vi "HandleAbort.vi"(8 "error in (no error)":errorcluster, 11 "Acquisition in":refnum<class "Acquisition.lvclass">) -> (0 "error out":errorcluster, 2 "abort?":bool, 3 "Acquisition out":refnum<class "Acquisition.lvclass">)   [LabVIEW 2018, in "Acquisition.lvclass"]
uses:
  Acquisition.lvclass
  C:/Users/devstaff/sparc4/s4gui/Versao ZeroMQ REQ-REP/SPARC4_GUI -v1.0.0/Server/Server.lvclass
  Server/Server.lvclass/Server.ctl
  Acquisition.lvclass/Acquisition.ctl
  Channel/Channel.lvclass
  StateMachine/State Machine.lvclass
  Server/Server.lvclass
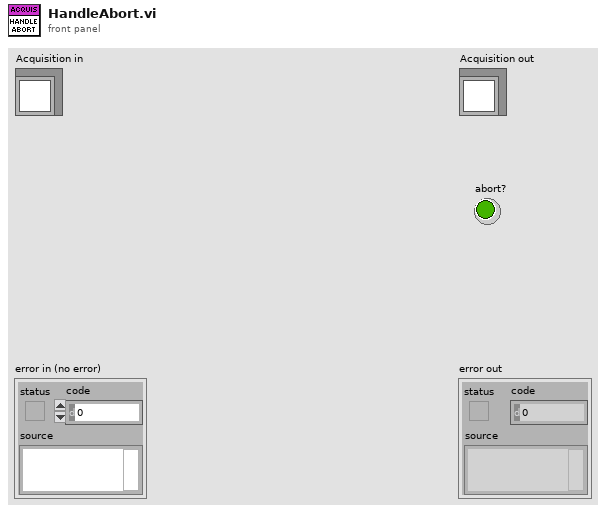
[diagram p1: front panel]
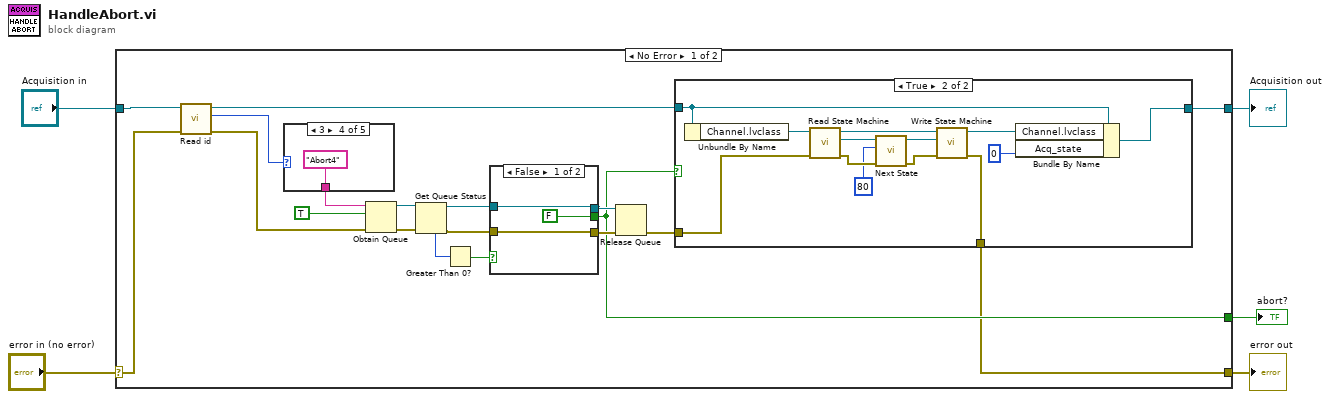
[diagram p0: block diagram]
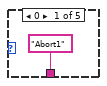
[diagram p2: hidden frame]
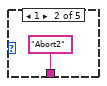
[diagram p3: hidden frame]
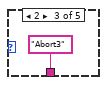
[diagram p4: hidden frame]
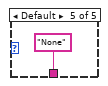
[diagram p5: hidden frame]
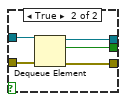
[diagram p7: hidden frame]
diagram:
  n1 = case shown="No Error" "error in (no error)" {
    selector: "error in (no error)" -> [w7 w54]
    tunnel: [w8 w54] -> w4
    tunnel: [w24 w53] -> w2
    tunnel: "Acquisition in" -> [w23 w53]
    tunnel: [w11 _] -> w1
    frame No Error {
      n2 = call "Read id.vi"("error in (no error)"=w7, "Server in"=w23) -> ("error out"=w6:errorcluster, "id"=w10:u32, "Server out"=w22:refnum<class "Acquisition.lvclass">)  [unwired: 7 in]
      n3 = case shown="3" w10 {
        tunnel: ["Abort1" ("name (unnamed)") "Abort2" ("name (unnamed)") "Abort3" ("name (unnamed)") "Abort4" ("name (unnamed)") "None" ("name (unnamed)")] -> w21
        frame 0 {
        }
        frame 1 {
        }
        frame 2 {
        }
        frame 3 {
        }
        frame Default {
        }
      }
      n4 = Obtain Queue(name (unnamed)=w21, element data type=TRUE, error in (no error)=w6) -> (queue out=w18:refnum<queue>, error out=w19:errorcluster)  [unwired: 2 in, 1 out]
      n5 = Get Queue Status(queue=w18, error in (no error)=w19) -> (queue out=w15:refnum<queue>, error out=w14:errorcluster, # elements in queue=w17:i32)  [unwired: 1 in, 5 out]
      n6 = Greater Than 0?(x=w17) -> (x > 0?=w16:bool)
      n7 = case shown="False" w16 {
        tunnel: w15 -> [w46 w51]
        tunnel: w14 -> [w45 w52]
        tunnel: [FALSE w50] -> w11
        tunnel: [w46 w49] -> w13
        tunnel: [w45 w48] -> w12
        frame False {
        }
        frame True {
          n8 = Dequeue Element(queue=w51, error in (no error)=w52) -> (queue out=w49:refnum<queue>, element=w50:bool, error out=w48:errorcluster)  [unwired: 1 in, 1 out]
        }
      }
      n9 = Release Queue(queue=w13, error in (no error)=w12) -> (error out=w9:errorcluster)  [unwired: 1 in, 2 out]
      n10 = case shown="True" w11 {
        tunnel: [w31 w35] -> w24
        tunnel: w22 -> [w31 w34]
        tunnel: w9 -> [w30 w33]
        tunnel: [w30 w32] -> w8
        frame False {
        }
        frame True {
          n11 = Unbundle By Name(w34) -> ("Channel.lvclass"=w37:refnum<class "Channel.lvclass">)
          n12 = call-dynamic "Read State Machine.vi"("error in (no error)"=w33, "Device in"=w37) -> ("error out"=w43:errorcluster, "State Machine.lvclass"=w44:refnum<class "State Machine.lvclass">, "Device out"=w41:refnum<class "Channel.lvclass">)  [unwired: 7 in]
          n13 = call "Next State.vi"("error in (no error)"=w43, "New_State"=u32 80, "State Machine in"=w44) -> ("error out"=w40:errorcluster, "State Machine out"=w42:refnum<class "State Machine.lvclass">)  [unwired: 7 in]
          n14 = call-dynamic "Write State Machine.vi"("error in (no error)"=w40, "State Machine.lvclass"=w42, "Device in"=w41) -> ("error out"=w32:errorcluster, "Device out"=w36:refnum<class "Channel.lvclass">)  [unwired: 7 in]
          n15 = Bundle By Name(cluster=w34, "Channel.lvclass"=w36, "Acq_state"=u32 0) -> (w35:refnum<class "Acquisition.lvclass">)
        }
      }
    }
    frame Error {
    }
  }
  "error out" <- w4
  "Acquisition out" <- w2
  "abort?" <- w1
